vi "LKIF2_SetTimingSync.vi"(8 "error in (no error)":errorcluster {"code" format="%x"}, 11 "OnOff":bool) -> (0 "error out":errorcluster {"code" format="%x"})   [LabVIEW 2013, in "Keyence LK-G5000.lvlib"]
uses:
  <instrlib>/Keyence LK-G5000/Keyence LK-G5000.lvlib
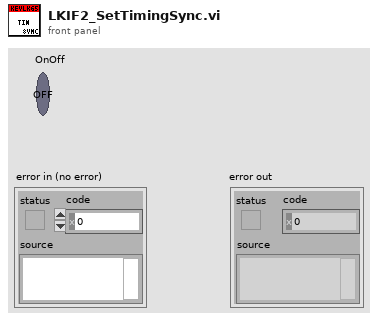
[diagram p1: front panel]
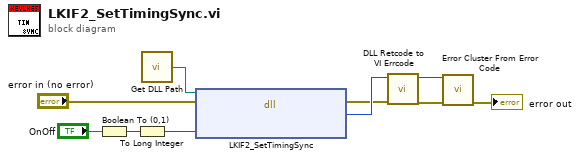
[diagram p0: block diagram]
diagram:
  n1 = Boolean To (0,1)(Boolean="OnOff") -> (0, 1=w6:i16)
  n2 = To Long Integer(number=w6) -> (32bit integer=w4:i32)
  n3 = call <instrlib>:"Get DLL Path.vi"() -> ("DLL Path"=w1:path)  [unwired: 1 in]
  n4 = dll-call lib="C:/Program Files/National Instruments/LabVIEW 2011/instr.lib/Keyence LK-G5000/LKIF2.dll" fn="LKIF2_SetTimingSync"(path in=w1, error in="error in (no error)", "OnOff"=w4) -> (error out=w2:errorcluster, "RC"=w3:i32)  [unwired: 2 in, 1 out]
  n5 = call <instrlib>:"DLL Retcode to VI Errcode.vi"("error in (no error)"=w2, "DLL Retcode"=w3) -> ("error out"=w10:errorcluster, "VI Errcode"=w9:i32)  [unwired: 8 in]
  n6 = call <vilib>:"Error Cluster From Error Code.vi"("error in (no error)"=w10, "error code (0)"=w9) -> ("error out"=→"error out":errorcluster)  [unwired: 7 in]
